vi "Add Column.vi"(6 "color":u32(colorbox)=16777215, 8 "error in":errorcluster, 9 "text":string, 10 "length":i32, 11 "XLS in":refnum<class "XLS.lvclass">) -> (0 "error out":errorcluster, 3 "XLS out":refnum<class "XLS.lvclass">)   [LabVIEW 2017, in "Report_lib.lvlib" / "XLS.lvclass"]
doc: "This method add colored row with some text\nin previously defined coordinates"
uses:
  XLS.lvclass
  XLS.lvclass/XLS.ctl
  <vilib>/Utility/NIReport.llb/Excel/NI_Excel.lvclass
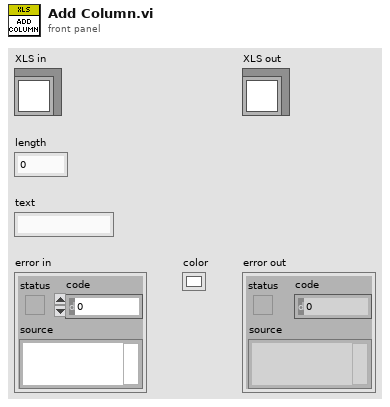
[diagram p1: front panel]
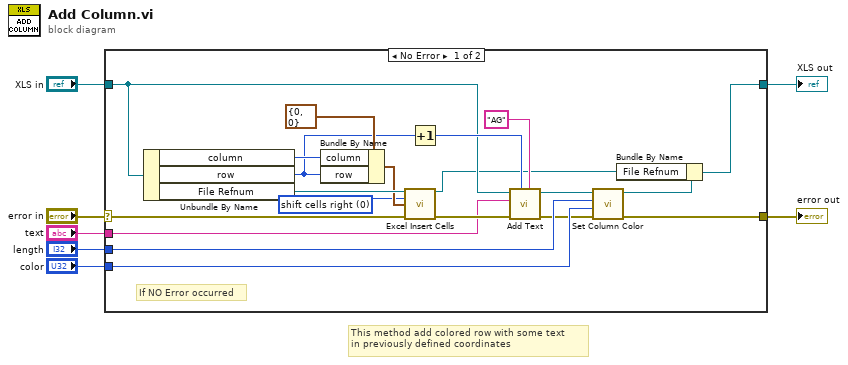
[diagram p0: block diagram]
diagram:
  # "This method add colored row with some text\nin previously defined coordinates"
  n1 = case shown="No Error" "error in" {
    selector: "error in" -> [w24 w29]
    tunnel: [w12 w29] -> w6
    tunnel: [w18 w28] -> w4
    tunnel: "XLS in" -> [w20 w28]
    tunnel: "text" -> [w17 _]
    tunnel: "length" -> [w15 _]
    tunnel: "color" -> [w14 _]
    frame No Error {
      w8 = u16 0 items=["shift cells right", "shift cells down", "entire row", "entire column"] ("mode (entire row)")
      # "If NO Error occurred"
      n2 = Unbundle By Name(w20) -> ("column"=w10:i32, "row"=w9:i32, "File Refnum"=w27:refnum<class "NI_report.lvclass">)
      n3 = Bundle By Name(cluster=cluster{"row":i32, "column":i32} {"row"=0, "column"=0} ("start (0, 0)"), "column"=w10, "row"=w9) -> (w25:cluster{"row":i32, "column":i32})
      n4 = call <vilib>:"Excel Insert Cells.vi"("report in"=w27, "mode (entire row)"=w8, "start (0, 0)"=w25, "error in (no error)"=w24) -> ("report out"=w19:refnum<class "NI_report.lvclass">, "error out"=w23:errorcluster)  [unwired: 10 in]
      n5 = Increment(x=w9) -> (x+1=w22:i32)
      n6 = call "Add Text.vi"("Adr"="AG", "Index"=w22, "error in"=w23, "text"=w17, "XLS in"=w20) -> ("error out"=w13:errorcluster, "XLS out"=w16:refnum<class "XLS.lvclass">)  [unwired: 5 in]
      n7 = call "Set Column Color.vi"("error in"=w13, "color"=w14, "length"=w15, "XLS in"=w16) -> ("error out"=w12:errorcluster, "XLS out"=w11:refnum<class "XLS.lvclass">)  [unwired: 6 in]
      n8 = Bundle By Name(cluster=w11, "File Refnum"=w19) -> (w18:refnum<class "XLS.lvclass">)
    }
    frame Error {
    }
  }
  "error out" <- w6
  "XLS out" <- w4
